vi "algo.host.test.create.algo.Watchlist.vi"() -> ()   [LabVIEW 2022 SP3]
panel:
  out "Passed":bool=TRUE
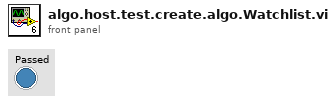
[diagram p1: front panel]
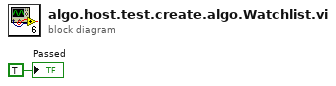
[diagram p0: block diagram]
diagram:
  "Passed" <- TRUE
